vi "Measurement Logic.vi"(8 "error in":errorcluster, 9 "measurement configuration":T13={"double array in"=[3.4, 5.6], "double in"=1.2, "U32 array in"=[32, 33], "U32 in"=32, "U64 array in"=[64, 65], "U64 in"=64, "I32 array in"=[-32, -33], "I32 in"=-32, "I64 array in"=[-64, -65], "I64 in"=-64, "bool in"=TRUE, "string in"="Lorem ipsum dolor sit", "u32 color ring in"=1, "u32 animal enum in"=enum."Gopher"} {"u32 color ring in" items=["Red", "Green", "Blue"]}, 10 "measure call context in":refnum<class "Measure Call Context.lvclass">) -> (0 "Error Out":errorcluster, 2 "measure call context out":refnum<class "Measure Call Context.lvclass">, 3 "measurement results":T1)   [LabVIEW 2025, in "Automotive Vision.lvclass"]
doc: "Contains the core logic for executing the measurement."
uses:
  Automotive Vision.lvclass
  1487 HIHO GSE/Host/Common/Types/Packet Table.ctl
  <vilib>/Plug-In SDKs/Measurements/Measure Call Context/Measure Call Context.lvclass
  Measurement Configuration.ctl
  <instrlib>/FlexRIO/CSI-2/v2/FPGA/Types/GPIO Bank.ctl
  <vilib>/userDefined/Silver/nirio_resource_slv.ctl
  1487 HIHO GSE/Host/Acq/Types/CSI-2 Data Source.ctl
  1487 HIHO GSE/Host/Common/Types/Serial Channel Configuration.ctl
  <instrlib>/FlexRIO/CSI-2/v2/FPGA/Types/Display Parameters.ctl
  <instrlib>/FlexRIO/CSI-2/v2/Common/Types/LLP Data Type.ctl
  1487 HIHO GSE/Host/Common/Types/RAW Interpretation for Display.ctl
  Measurement Results.ctl
  <instrlib>/FlexRIO/CSI-2/v2/FPGA/Types/Timestamp ID.ctl
  1487 HIHO GSE/Host/Common/Types/GPIO Filter.ctl
  1487 HIHO GSE/FPGA/Common/Types/SerDes Identifier.ctl
  <vilib>/vision/Image Controls.llb/IMAQ Image.ctl
  <vilib>/Utility/miscctls.llb/LVRowAndColumnUnsignedTypeDef.ctl
  <instrlib>/FlexRIO/API/Host/v1/NI FlexRIO/API/Wait for PoC Safe to Disconnect Channels Array.vi
  <vilib>/FPGAPlugInAG/Dynamic/niLvFpga_Close_Dynamic.vi
  <extravilib>/ChannelInstances/Event Messenger-bool/Instantiate.vi
  <vilib>/rvi/interface/nirviCloseFPGA/nirviCloseFPGA.xnode
  Automotive Vision.lvclass/Automotive Vision.ctl
  1487 HIHO GSE/Host/Acq/GettingStarted_Acq_148X_Host.lvlib
  1487 HIHO GSE/Host/Common/GettingStarted_Common_148X_Host.lvlib
  <instrlib>/FlexRIO/API/Host/v1/NI FlexRIO API v1.lvlib
  <instrlib>/FlexRIO/CSI-2/v2/Common/NI CSI-2 API Common v2.lvlib
  <instrlib>/FlexRIO/CSI-2/v2/FPGA/NI CSI-2 API FPGA v2.lvlib
  1487 HIHO GSE/FPGA/Common/GettingStarted_Common_148X_FPGA.lvlib
panel:
  in  "Array":u32[](array[numeric])
  in  "Serial Channel (2nd Display)":fxp<+,3,3>
  in  "Serial Channel (1st Display)":fxp<+,3,3>
  in  "Configuration":T2(tab)
  in  "TDMS File Directory":path=path "C:/dev/hardware-validation/src/labview/auto-vision/Automotive Vision/1487 HIHO GSE/TDMS capture"
  in  "RIO Device":T3="PXI1Slot2"
  in  "Channel Configurations":T4[](array[typedef])=[{"Serial Channel"="SI1", "FPGA Display Parameters"={"virtual channel"=0.0, "payload data type"=enum."RAW 8", "frame skip count"=0, "line skip count"=0, "pixel skip count"=0.0}, "RAW Display Parameters"={"Interpretation"=enum."Bayer", "Bayer Parameters"={"Pattern"=3, "Algorithm"=0, "Red Gain"=1.0, "Green Gain"=1.0, "Blue Gain"=1.0}}}] {"RAW Display Parameters"."Bayer Parameters"."Blue Gain" min=0.0 max=3.99 step=0.1 format="%_4g"; "RAW Display Parameters"."Bayer Parameters"."Green Gain" min=0.0 max=3.99 step=0.1 format="%_4g"; "RAW Display Parameters"."Bayer Parameters"."Red Gain" min=0.0 max=3.99 step=0.1 format="%_4g"; "RAW Display Parameters"."Bayer Parameters"."Algorithm" items=["Bilinear", "VNG"]; "RAW Display Parameters"."Bayer Parameters"."Pattern" items=["GB", "GR", "BG", "RG"]}
  in  "CSI-2 Data Source":T8=1 items=["Raw", "Corrected"]
  in  "Configuration Script":path=path "C:/dev/hardware-validation/src/labview/auto-vision/Automotive Vision/1487 HIHO GSE/scripts/Image Receiver Scripts/9296A_RAW8.cpp"
  in  "Serial Input Active Lane Count":i32(ring)=4 items=["1 Lane"=1, "2 Lanes"=2, "4 Lanes"=4]
  in  "Reference Clock Frequency (Hz)":dbl=25000000.0 format="%#_6p"
  in  "Power Over Coax Source":i32(ring) items=["None", "Internal", "Auxiliary"]
  out "GPIO Bank Read":T9
  out "Power Over Coax Voltage (V)":dbl[](array[numeric]) format="%#.2pV"
  out "Power Over Coax Current (A)":dbl[](array[numeric]) format="%#.2pA"
  in  "Acquired Serial Input Channel Data":T10(tab)
  out "Source Rate (fps)(1st Display)":dbl
  out "Update Rate (fps)(1st Display)":dbl
  out "1st channel display":T11(plugin-control)
  out "Bytes Acquired (1st Channel)":i64 format="%#.6p"
  out "Source Rate (fps)(2nd Display)":dbl
  out "Update Rate (fps)(2nd Display)":dbl
  out "2nd channel display":T11(plugin-control)
  out "Acquired Packets (1st Channel)":T12
  out "Packets Logged (1st Channel)":i64
  out "Bytes Acquired (2nd Channel)":i64 format="%#.6p"
  out "Acquired Packets (2nd Channel)":T12
  out "Packets Logged (2nd Channel)":i64
  out "I2C Timestamps":T12
  out "GPIO Timestamps Waveform":digitalwaveform[](graph)
  out "Error Parsing GPIO Timestamps":bool
  out "Power Over Coax Source In Range":bool[](array[boolean])
  in  "Stop Acquisition":bool
  out "Acquisition In Progress":bool
  out "Acquisition Duration (s) 2":dbl format="%.1f"
  out "Acquisition Stopped":bool
  # "Resource Configuration"
  # "Data Output Configuration"
  # "Channel Configuration"
  # "Acquisition Configuration"
  # "First and Last Packet Select Configuration"
  # "Packet Filter Configuration"
  # "Power Over Coax Configuration"
  # "Clocking Configuration"
  # "I2C Timestamp Configuration"
  # "The timestamp filters listed correspond to the I2C traffic for a specific serial channel:\n\nUser24 = SI0\nUser25 = SI1\nUser26 = SI2\nUser27 = SI3\nUser28 = SI4\nUser29 = SI5\nUser30 = SI6\nUser31 = SI7"
  # "GPIO Configuration"
  # "* For additional packet viewing capability, use GettingStarted_Common_148X_Host.lvlib->TDMS File Viewer.vi"
  # "* For additional packet viewing capability, use GettingStarted_Common_148X_Host.lvlib->TDMS File Viewer.vi"
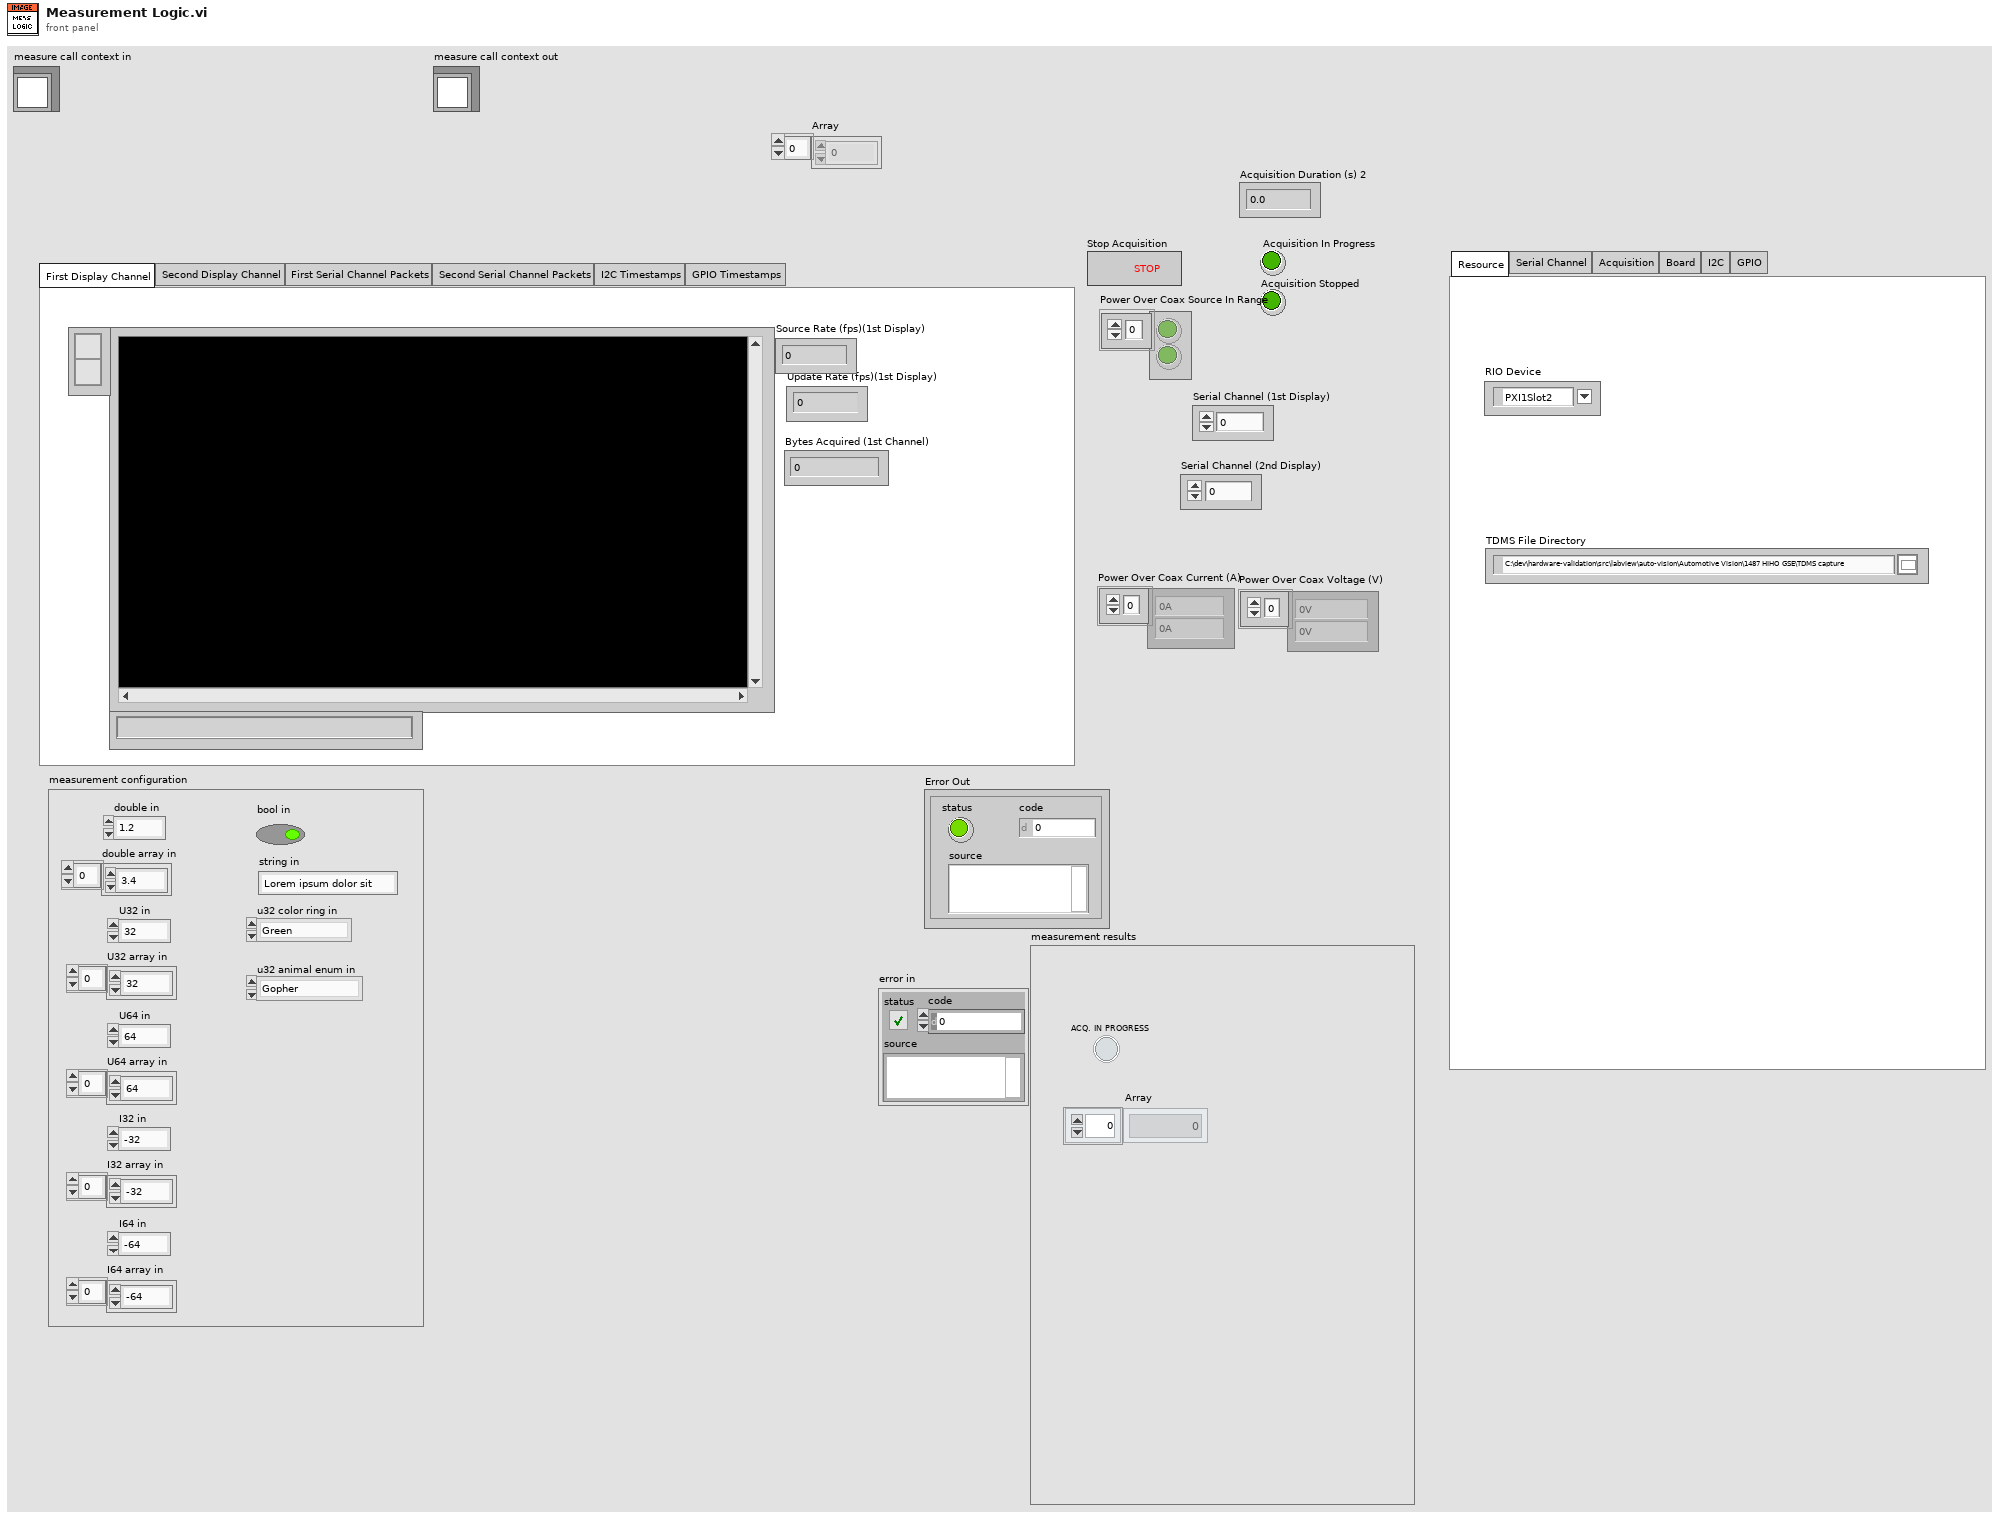
[diagram p1: front panel]
types:
  T1 = typedef "Automotive Vision.lvclass/Measurement Results.ctl" = cluster{"ACQ. IN PROGRESS":bool, "Array":u32[]}
  T2 = enum32{"Resource", "Serial Channel", "Acquisition", "Board", "I2C", "GPIO"}
  T3 = typedef "nirio_resource_slv.ctl" = tag
  T4 = typedef "GettingStarted_Common_148X_Host.lvlib/Serial Channel Configuration.ctl" = cluster{"Serial Channel":string, "FPGA Display Parameters":T5, "RAW Display Parameters":cluster{"Interpretation":T7, "Bayer Parameters":cluster{"Pattern":i32, "Algorithm":i32, "Red Gain":dbl, "Green Gain":dbl, "Blue Gain":dbl}}}
  T5 = typedef "NI CSI-2 API FPGA v2.lvlib/Display Parameters.ctl" = cluster{"virtual channel":fxp<+,4,4>, "payload data type":T6, "frame skip count":u16, "line skip count":u8, "pixel skip count":fxp<+,5,5>}
  T6 = typedef "NI CSI-2 API Common v2.lvlib/LLP Data Type.ctl" = enum8{"Frame Start", "Frame End", "Line Start", "Line End", "End of Transmission", "Reserved 0", "Reserved 1", "Reserved 2", "Generic Short Packet 1", "Generic Short Packet 2", "Generic Short Packet 3", "Generic Short Packet 4", "Generic Short Packet 5", "Generic Short Packet 6", "Generic Short Packet 7", "Generic Short Packet 8", "Null", "Blanking Data", "Embedded 8-bit non Image Data", "Generic Long Packet 1", "Generic Long Packet 2", "Generic Long Packet 3", "Generic Long Packet 4", "Reserved 3", "YUV420 8-bit", "YUV420 10-bit", "Legacy YUV420 8-bit", "Reserved 4", "YUV420 8-bit Chroma Shifted", "YUV420 10-bit Chroma Shifted", "YUV422 8-bit", "YUV422 10-bit", "RGB444", "RGB555", "RGB565", "RGB666", "RGB888", "Reserved 5", "Reserved 6", "RAW 24", "RAW 6", "RAW 7", "RAW 8", "RAW 10", "RAW 12", "RAW 14", "RAW 16", "RAW 20", "User Defined 8-bit Data 1", "User Defined 8-bit Data 2", "User Defined 8-bit Data 3", "User Defined 8-bit Data 4", "User Defined 8-bit Data 5", "User Defined 8-bit Data 6", "User Defined 8-bit Data 7", "User Defined 8-bit Data 8", "USL Command", "Reserved 7", "Reserved 8", "Reserved 9", "Reserved 10", "Reserved 11", "Reserved 12", "LRTE EPD Spacer"}
  T7 = typedef "GettingStarted_Common_148X_Host.lvlib/RAW Interpretation for Display.ctl" = enum16{"Grayscale", "Bayer", "RGB", "YUV422", "YUV420", "Legacy YUV420"}
  T8 = typedef "GettingStarted_Acq_148X_Host.lvlib/CSI-2 Data Source.ctl" = u16
  T9 = typedef "NI CSI-2 API FPGA v2.lvlib/GPIO Bank.ctl" = cluster{"GPIO 0":bool, "GPIO 1":bool, "GPIO 2":bool, "GPIO 3":bool, "GPIO 4":bool, "GPIO 5":bool, "GPIO 6":bool, "GPIO 7":bool, "GPIO 8":bool, "GPIO 9":bool, "GPIO 10":bool}
  T10 = enum32{"First Display Channel", "Second Display Channel", "First Serial Channel Packets", "Second Serial Channel Packets", "I2C Timestamps", "GPIO Timestamps"}
  T11 = typedef "IMAQ Image.ctl" = refnum<image>
  T12 = typedef "GettingStarted_Common_148X_Host.lvlib/Packet Table.ctl" = string[][]
  T13 = typedef "Automotive Vision.lvclass/Measurement Configuration.ctl" = cluster{"double array in":dbl[], "double in":dbl, "U32 array in":u32[], "U32 in":u32, "U64 array in":u64[], "U64 in":u64, "I32 array in":i32[], "I32 in":i32, "I64 array in":i64[], "I64 in":i64, "bool in":bool, "string in":string, "u32 color ring in":u32, "u32 animal enum in":enum32{"Rabbit", "Gopher", "Badger"}}
  T14 = typedef "GettingStarted_Common_148X_Host.lvlib/GPIO Filter.ctl" = cluster{"GPIO Bank":T15, "GPIO Number":i32}
  T15 = typedef "NI CSI-2 API FPGA v2.lvlib/Timestamp ID.ctl" = enum8{"SI0 LLP", "SI1 LLP", "SI2 LLP", "SI3 LLP", "SI4 LLP", "SI5 LLP", "SI6 LLP", "SI7 LLP", "SO0 LLP", "SO1 LLP", "SO2 LLP", "SO3 LLP", "SO4 LLP", "SO5 LLP", "SO6 LLP", "SO7 LLP", "Ser0 GPIO Bank", "Ser1 GPIO Bank", "Ser2 GPIO Bank", "Ser3 GPIO Bank", "Ser4 GPIO Bank", "Ser5 GPIO Bank", "Ser6 GPIO Bank", "Ser7 GPIO Bank", "Des0 GPIO Bank", "Des1 GPIO Bank", "Des2 GPIO Bank", "Des3 GPIO Bank", "Des4 GPIO Bank", "Des5 GPIO Bank", "Des6 GPIO Bank", "Des7 GPIO Bank", "User0", "User1", "User2", "User3", "User4", "User5", "User6", "User7", "User8", "User9", "User10", "User11", "User12", "User13", "User14", "User15", "User16", "User17", "User18", "User19", "User20", "User21", "User22", "User23", "User24", "User25", "User26", "User27", "User28", "User29", "User30", "User31"}
  T16 = typedef "LVRowAndColumnUnsignedTypeDef.ctl" = cluster{"Row":u32, "Column":u32}
  T17 = typedef "GettingStarted_Common_148X_Host.lvlib/Serial Channel Display Parameters.ctl" = cluster{"images":cluster{"grayscale":T11, "color":T11}, "RAW parameters":cluster{"interpretation":T7, "bayer parameters":cluster{"pattern":i32, "algorithm":i32, "red gain":dbl, "green gain":dbl, "blue gain":dbl}}}
  T18 = cluster{"Source Rate (fps)(1st Display)":refnum<vi>, "Update Rate (fps)(1st Display)":refnum<vi>}
  T19 = cluster{"Source Rate (fps)(2nd Display)":refnum<vi>, "Update Rate (fps)(2nd Display)":refnum<vi>}
  T20 = cluster{"Source Rate (fps)(2nd Display)":refnum<vi>, "Update Rate (fps)(2nd Display)":refnum<vi>}[]
  T21 = typedef "GettingStarted_Common_148X_FPGA.lvlib/SerDes Identifier.ctl" = enum8{"None", "SI 0 Deserializer", "SI 1 Deserializer", "SI 2 Deserializer", "SI 3 Deserializer", "SI 4 Deserializer", "SI 5 Deserializer", "SI 6 Deserializer", "SI 7 Deserializer", "SO 0 Serializer", "SO 1 Serializer", "SO 2 Serializer", "SO 3 Serializer", "SO 4 Serializer", "SO 5 Serializer", "SO 6 Serializer", "SO 7 Serializer", "SI 0 SI 1 Deserializer", "SI 2 SI 3 Deserializer", "SI 4 SI 5 Deserializer", "SI 6 SI 7 Deserializer"}
  T22 = typedef "Event Messenger-bool.lvlib/))Channel.ctl" = refnum<queue>
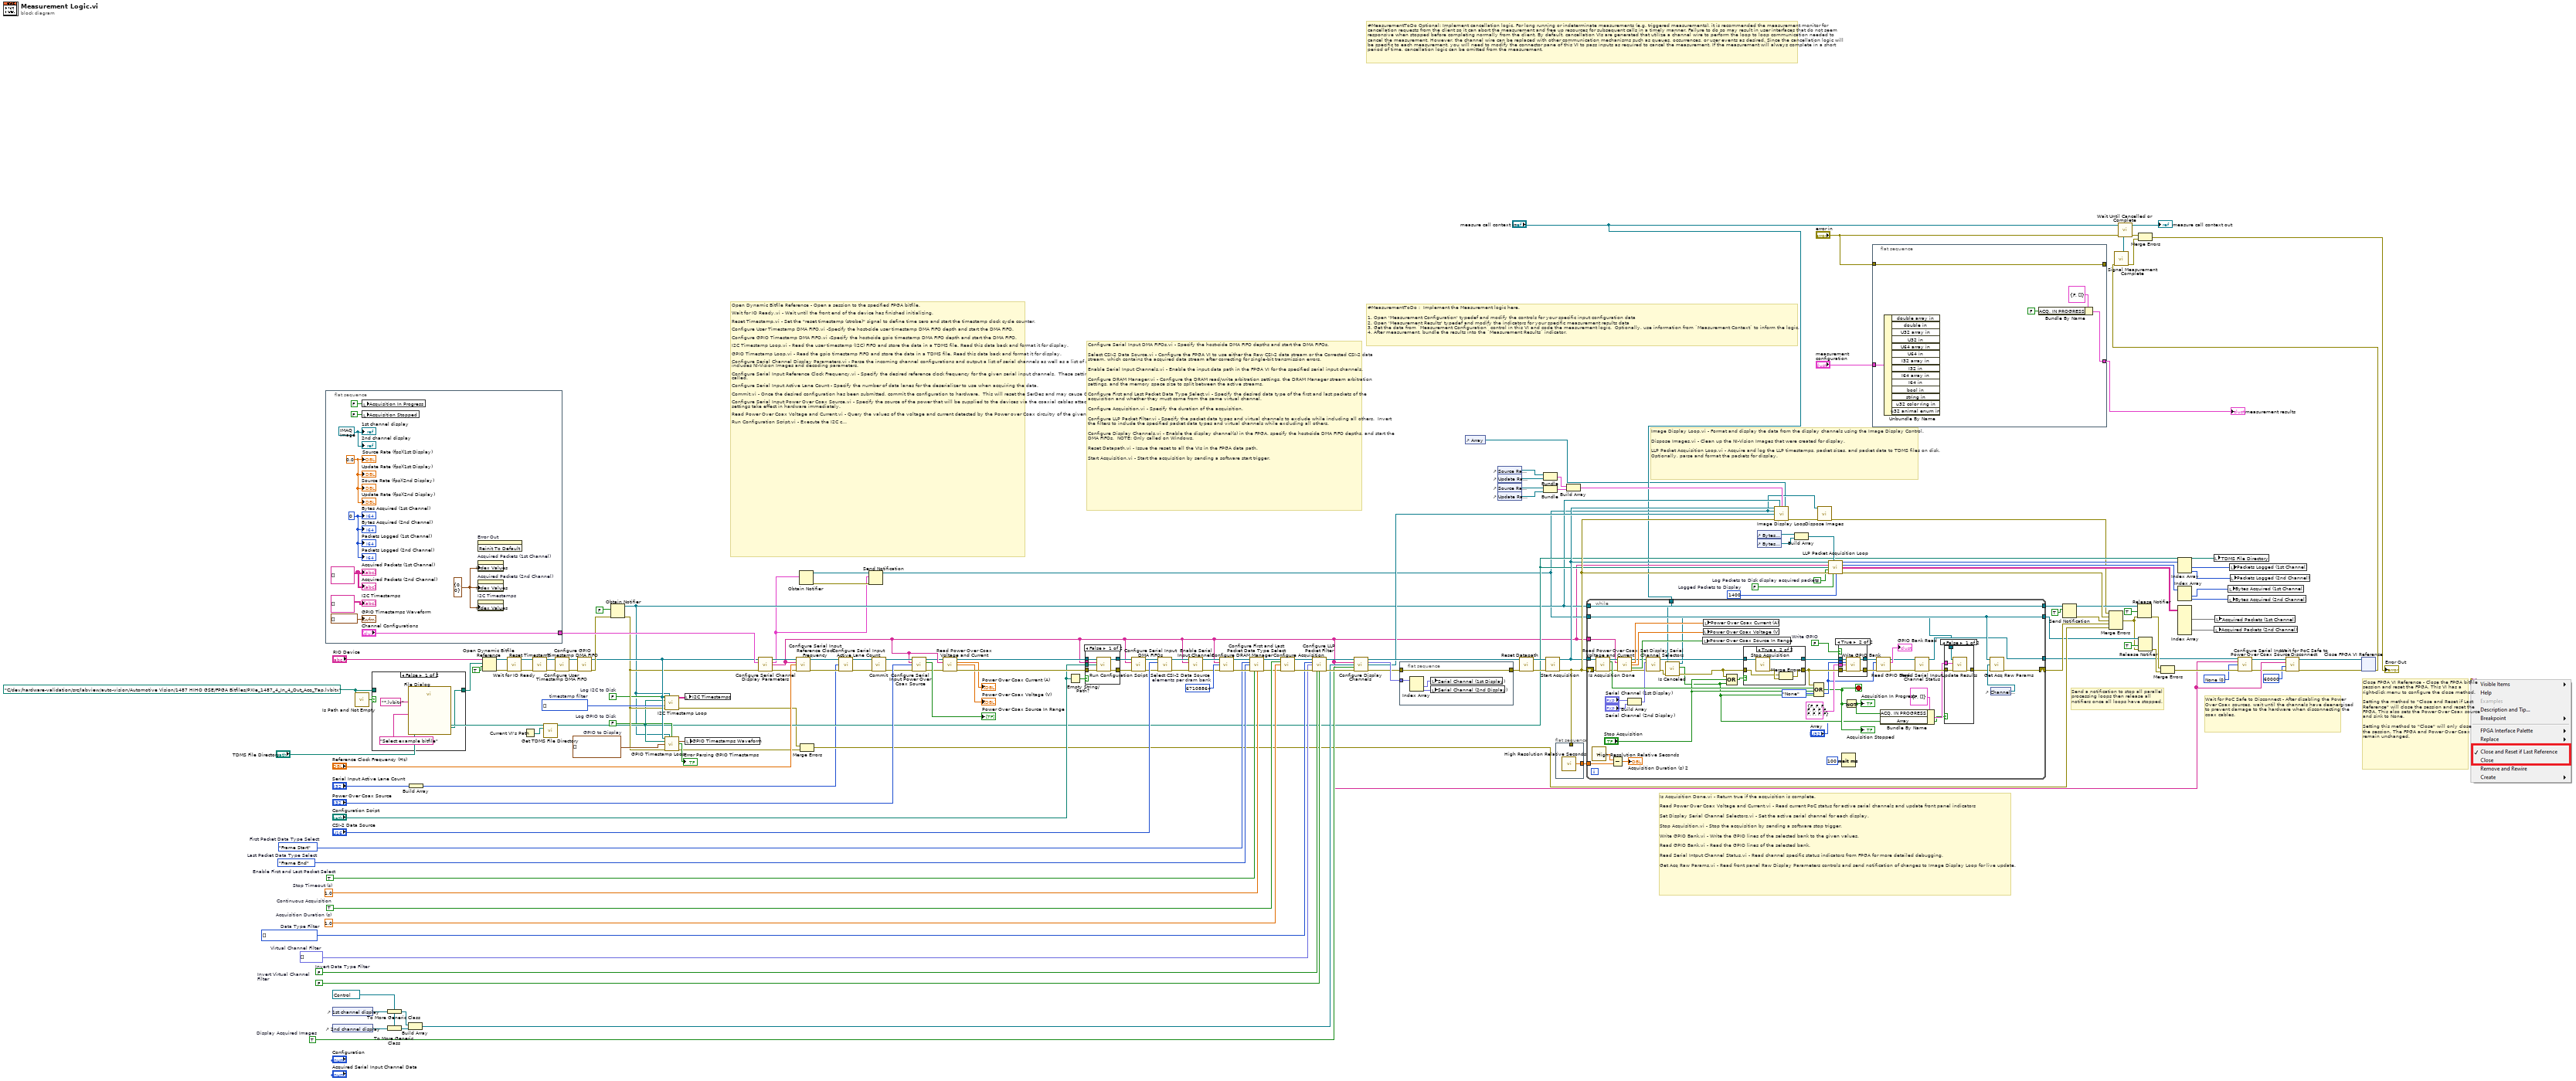
[diagram p0: block diagram]
diagram:
  w35 = i64 1400  # Logged Packets to Display
  w74 = FALSE  # Log Packets to Disk
  w123 = FALSE  # Invert Virtual Channel Filter
  w124 = FALSE  # Invert Data Type Filter
  w130 = fxp<+,4,4>[] []  # Virtual Channel Filter
  w45 = T14[] []  # GPIO to Display
  w41 = FALSE  # Log GPIO to Disk
  w44 = T15[] [] items=["SI0 LLP", "SI1 LLP", "SI2 LLP", "SI3 LLP", "SI4 LLP", "SI5 LLP", "SI6 LLP", "SI7 LLP", "SO0 LLP", "SO1 LLP", "SO2 LLP", "SO3 LLP", "SO4 LLP", "SO5 LLP", "SO6 LLP", "SO7 LLP", "Ser0 GPIO Bank", "Ser1 GPIO Bank", "Ser2 GPIO Bank", "Ser3 GPIO Bank", "Ser4 GPIO Bank", "Ser5 GPIO Bank", "Ser6 GPIO Bank", "Ser7 GPIO Bank", "Des0 GPIO Bank", "Des1 GPIO Bank", "Des2 GPIO Bank", "Des3 GPIO Bank", "Des4 GPIO Bank", "Des5 GPIO Bank", "Des6 GPIO Bank", "Des7 GPIO Bank", "User0", "User1", "User2", "User3", "User4", "User5", "User6", "User7", "User8", "User9", "User10", "User11", "User12", "User13", "User14", "User15", "User16", "User17", "User18", "User19", "User20", "User21", "User22", "User23", "User24", "User25", "User26", "User27", "User28", "User29", "User30", "User31"]  # timestamp filter
  w42 = FALSE  # Log I2C to Disk
  w69 = TRUE  # Display Acquired Images
  w137 = T6[] [] items=["Frame Start", "Frame End", "Line Start", "Line End", "End of Transmission", "Reserved 0", "Reserved 1", "Reserved 2", "Generic Short Packet 1", "Generic Short Packet 2", "Generic Short Packet 3", "Generic Short Packet 4", "Generic Short Packet 5", "Generic Short Packet 6", "Generic Short Packet 7", "Generic Short Packet 8", "Null", "Blanking Data", "Embedded 8-bit non Image Data", "Generic Long Packet 1", "Generic Long Packet 2", "Generic Long Packet 3", "Generic Long Packet 4", "Reserved 3", "YUV420 8-bit", "YUV420 10-bit", "Legacy YUV420 8-bit", "Reserved 4", "YUV420 8-bit Chroma Shifted", "YUV420 10-bit Chroma Shifted", "YUV422 8-bit", "YUV422 10-bit", "RGB444", "RGB555", "RGB565", "RGB666", "RGB888", "Reserved 5", "Reserved 6", "RAW 24", "RAW 6", "RAW 7", "RAW 8", "RAW 10", "RAW 12", "RAW 14", "RAW 16", "RAW 20", "User Defined 8-bit Data 1", "User Defined 8-bit Data 2", "User Defined 8-bit Data 3", "User Defined 8-bit Data 4", "User Defined 8-bit Data 5", "User Defined 8-bit Data 6", "User Defined 8-bit Data 7", "User Defined 8-bit Data 8", "USL Command", "Reserved 7", "Reserved 8", "Reserved 9", "Reserved 10", "Reserved 11", "Reserved 12", "LRTE EPD Spacer"]  # Data Type Filter
  w140 = 1.0  # Acquisition Duration (s)
  w146 = TRUE  # Continuous Acquisition
  w112 = 1.0  # Stop Timeout (s)
  w113 = TRUE  # Enable First and Last Packet Select
  w110 = LLP_Data_Type."Frame End"  # Last Packet Data Type Select
  w111 = LLP_Data_Type."Frame Start"  # First Packet Data Type Select
  w135 = path "C:/dev/hardware-validation/src/labview/auto-vision/Automotive Vision/1487 HIHO GSE/FPGA Bitfiles/PXIe_1487_4_In_4_Out_Acq_Tap.lvbitx" ("Bitfile Path")
  w9 = 0 items=["None", "Internal", "Auxiliary"] ("power over coax source")
  w36 = TRUE  # display acquired packets
  w87 = refnum<vi> refnum ("image display reference")
  w152 = u32 67108864  # elements per dram bank
  # "Wait for PoC Safe to Disconnect - After disabling the Power Over Coax sources, wait until the channels have deenergized to prevent damage to the hardware when disconnecting the coax cables."
  # "Send a notification to stop all parallel processing loops then release all notifiers once all loops have stopped."
  # "Image Display Loop.vi - Format and display the data from the display channels using the Image Display Control.   \n\nDispose Images.vi - Clean up the NI-Vision Images that were created for display.\n\nLLP Packet Acquisition Loop.vi - Acquire and log the LLP timestamps, packet sizes, and packet data to TDMS files on disk.  Optionally, parse and format the packets for display."
  # "Configure Serial Input DMA FIFOs.vi - Specify the host-side DMA FIFO depths and start the DMA FIFOs.\n\nSelect CSI-2 Data Source.vi - Configure the FPGA VI to use either the Raw CSI-2 data stream or the Corrected CSI-2 data stream, which contains the acquired data stream after correcting for single-bit transmission errors.\n\nEnable Serial Input Channels.vi - Enable the input data path in the FPGA VI for the specified serial input channels.\n\nConfigure DRAM Manager.vi - Configure the DRAM read/write arbitration settings, the DRAM Manager stream arbitration settings, and the memory space size to split between the active streams.\n\nConfigure First and Last Packet Data Type Select.vi - Specify the desired data type of the first and last packets of the acquisition and whether they must come from the same virtual channel.\n\nConfigure Acquisition.vi - Specify the duration of the acquisition.\n\nConfigure LLP Packet Filter.vi - Specify the packet data types and virtual channels to exclude while including all others.  Invert the filters to include the specified packet data types and virtual channels while excluding all others.\n\nConfigure Display Channels.vi - Enable the display channel(s) in the FPGA, specify the host-side DMA FIFO depths, and start the DMA FIFOs.  NOTE: Only called on Windows. \n\nReset Datapath.vi - Issue the reset to all the VIs in the FPGA data path.\n\nStart Acquisition.vi - Start the acquisition by sending a software start trigger."
  # "Close FPGA VI Reference - Close the FPGA bitfile session and reset the FPGA. This VI has a right-click menu to configure the close method. \n\nSetting the method to \"Close and Reset if Last Reference\" will close the session and reset the FPGA. This also sets the Power Over Coax source and sink to None.\n\nSetting this method to \"Close\" will only close the session. The FPGA and Power Over Coax remain unchanged."
  # "Open Dynamic Bitfile Reference - Open a session to the specified FPGA bitfile.\n\nWait for IO Ready.vi - Wait until the front end of the device has finished initializing.\n\nReset Timestamp.vi - Set the \"reset timestamp (strobe)\" signal to define time zero and start the timestamp clock cycle counter.\n\nConfigure User Timestamp DMA FIFO.vi -Specify the host-side user timestamp DMA FIFO depth and start the DMA FIFO.\n\nConfigure GPIO Timestamp DMA FIFO.vi -Specify the host-side gpio timestamp DMA FIFO depth and start the DMA FIFO.\n\nI2C Timestamp Loop.vi - Read the user timestamp (I2C) FIFO and store the data in a TDMS file. Read this data back and format it for display.\n\nGPIO Timestamp Loop.vi - Read the gpio timestamp FIFO and store the data in a TDMS file. Read this data back and format it for display.\n\nConfigure Serial Channel Display Parameters.vi - Parse the incoming channel configurations and output a list of serial channels as well as a list of serial channel display parameters, which includes NI-Vision Images and decoding parameters.\n\nConfigure Serial Input Reference Clock Frequency.vi - Specify the desired reference clock frequency for the given serial input channels.  These settings do not take effect until Commit.vi is called.\n\nConfigure Serial Input Active Lane Count - Specify the number of data lanes for the deserializer to use when acquiring the data. \n\nCommit.vi - Once the desired configuration has been submitted, commit the configuration to hardware.  This will reset the SerDes and may cause GPIO lines to toggle. \n\nConfigure Serial Input Power Over Coax Source.vi - Specify the source of the power that will be supplied to the devices via the coaxial cables attached to the given serial input channels.  These settings take effect in hardware immediately.\n\nRead Power Over Coax Voltage and Current.vi - Query the values of the voltage and current detected by the Power over Coax circuitry of the given serial channels.\n\nRun Configuration Script.vi - Execute the I2C commands in the specified script file for the given serial channels.  The script is used to configure the serializer, deserializer, or other I2C slave device, such as the image sensor."
  # "Is Acquisition Done.vi - Return true if the acquisition is complete.\n\nRead Power Over Coax Voltage and Current.vi - Read current PoC status for active serial channels and update front panel indicators \n\nSet Display Serial Channel Selectors.vi - Set the active serial channel for each display.\n\nStop Acquisition.vi - Stop the acquisition by sending a software stop trigger.\n\nWrite GPIO Bank.vi - Write the GPIO lines of the selected bank to the given values.\n\nRead GPIO Bank.vi - Read the GPIO lines of the selected bank.\n\nRead Serial Intput Channel Status.vi - Read channel specific status indicators from FPGA for more detailed debugging.\n\nGet Acq Raw Params.vi - Read front panel Raw Display Parameters controls and send notification of changes to Image Display Loop for live update."
  # "#MeasurementToDo Optional: Implement cancellation logic. For long running or indeterminate measurements (e.g. triggered measurements), it is recommended the measurement monitor for cancellation requests from the client so it can abort the measurement and free up resources for subsequent calls in a timely manner. Failure to do so may result in user interfaces that do not seem responsive when stopped before completing normally from the client. By default, cancellation VIs are generated that utilize a channel wire to perform the loop to loop communication needed to cancel the measurement. However, the channel wire can be replaced with other communication mechanisms such as queues, occurrences, or user events as desired. Since the cancellation logic will be specific to each measurement, you will need to modify the connector pane of this VI to pass inputs as required to cancel the measurement. If the measurement will always complete in a short period of time, cancellation logic can be omitted from the measurement."
  # "#MeasurementToDo :  Implement the Measurement logic here.\n\n1. Open 'Measurement Configuration' typedef and modify the controls for your specific input configuration data\n2. Open 'Measurement Results' typedef and modify the indicators for your specific measurement results data\n3. Get the data from `Measurement Configuration` control in this VI and code the measurement logic.  Optionally, use information from `Measurement Context` to inform the logic.\n4. After measurement, bundle the results into the `Measurement Results` indicator."
  n1 = flat-sequence {
    tunnel: ["Channel Configurations"] -> w101
    frame #0 {
      w159 = T16 {"Row"=0, "Column"=0} ("Index Values")
      w166 = T12 [] ("Acquired Packets (1st Channel)")
      w162 = 0 ("Number of Packets Acquired (1st Channel)")
      w165 = 0.0 ("display fps (2nd display)")
      w168 = T11 refnum ("first channel display")
      n2 = local write "Acquisition In Progress"(FALSE ("Acquisition In Progress")) -> ()
      n3 = local write "Acquisition Stopped"(FALSE ("Acquisition Stopped")) -> ()
      n4 = invoke on="Error Out" class="Clust (strict)" method="Reinit To Default"() -> ()  [unwired: 3 in, 3 out]
      n5 = property on="Acquired Packets (1st Channel)" class="Tbl (strict)"("Index Values"=w159) -> ()  [unwired: 2 in, 2 out]
      n6 = property on="Acquired Packets (2nd Channel)" class="Tbl (strict)"("Index Values"=w159) -> ()  [unwired: 2 in, 2 out]
      n7 = property on="I2C Timestamps" class="Tbl (strict)"("Index Values"=w159) -> ()  [unwired: 2 in, 2 out]
      "1st channel display" <- w168
      "2nd channel display" <- w168
      "Update Rate (fps)(1st Display)" <- w165
      "Update Rate (fps)(2nd Display)" <- w165
      "Acquired Packets (1st Channel)" <- w166
      "Packets Logged (1st Channel)" <- w162
      "Acquired Packets (2nd Channel)" <- w166
      "Packets Logged (2nd Channel)" <- w162
      "Source Rate (fps)(1st Display)" <- w165
      "Source Rate (fps)(2nd Display)" <- w165
      "GPIO Timestamps Waveform" <- digitalwaveform[] [] ("GPIO Timestamps Waveform")
      "I2C Timestamps" <- T12 [] ("I2C Timestamps 2")
      "Bytes Acquired (1st Channel)" <- w162
      "Bytes Acquired (2nd Channel)" <- w162
    }
  }
  n8 = control-ref of="1st channel display"() -> (w98:refnum<vi>)
  n9 = control-ref of="2nd channel display"() -> (w96:refnum<vi>)
  n10 = call <vilib>:"Is Path and Not Empty.vi"("path"=w135) -> ("Is Path and Not Empty?"=w134:bool)  [unwired: 4 in]
  n11 = case shown="False" w134 {
    tunnel: w135 -> [_ w172]
    tunnel: [w170 w172] -> w133
    frame False {
      n12 = call "File Dialog"("prompt"="Select example bitfile", "pattern (all files)"="*.lvbitx") -> ("selected path"=w170:path)  [unwired: 10 in, 3 out]
    }
    frame True {
    }
  }
  n13 = To More Generic Class(target class=w87, reference=w98) -> (generic class reference=w97:refnum<vi>)
  n14 = To More Generic Class(target class=w87, reference=w96) -> (generic class reference=w95:refnum<vi>)
  n15 = Build Array(w97, w95) -> (w93:refnum<vi>[])
  n16 = Build Array("Serial Input Active Lane Count") -> (w27:i32[])
  n17 = Open Dynamic Bitfile Reference(0:"RIO Device", 1:w133, 2:TRUE ("Run When Loaded")) -> (5:w131:refnum<k20>, 8:w132:errorcluster)  [unwired: 2 in]
  n18 = call <instrlib>:"Wait for IO Ready.vi"("fpga interface in"=w131, "error in"=w132) -> ("fpga interface out"=w65:refnum<k20>, "error out"=w66:errorcluster)  [unwired: 10 in, 2 out]
  n19 = Current VI's Path() -> (path=w105:path)
  n20 = call "Reset Timestamp.vi"("fpga interface in"=w65, "error in (no error)"=w66) -> ("fpga interface out"=w55:refnum<k20>, "error out"=w54:errorcluster)  [unwired: 12 in]
  n21 = call "Get TDMS File Directory.vi"("tdms file directory in"="TDMS File Directory", "calling vi path"=w105) -> ("tdms file directory out"=w40:path)  [unwired: 13 in]
  n22 = call "Configure User Timestamp DMA FIFO.vi"("fpga interface in"=w55, "error in (no error)"=w54) -> ("fpga interface out"=w53:refnum<k20>, "error out"=w52:errorcluster)  [unwired: 12 in]
  n23 = call "Configure GPIO Timestamp DMA FIFO.vi"("fpga interface in"=w53, "error in (no error)"=w52) -> ("fpga interface out"=w49:refnum<k20>, "error out"=w51:errorcluster)  [unwired: 12 in]
  n24 = Obtain Notifier(notification data type=FALSE ("result"), error in (no error)=w51) -> (notifier out=w26:refnum<notifier>, error out=w43:errorcluster)  [unwired: 2 in, 1 out]
  n25 = call "I2C Timestamp Loop.vi"("fpga interface in"=w49, "'stop' notifier"=w26, "log i2c to disk"=w42, "tdms file directory"=w40, "timestamp filter"=w44, "error in (no error)"=w43) -> ("i2c data"=w48:string[][], "error out"=w38:errorcluster)  [unwired: 8 in]
  n26 = call "GPIO Timestamp Loop.vi"("fpga interface in"=w49, "'stop' notifier"=w26, "log gpio to disk"=w41, "tdms file directory"=w40, "gpio to display"=w45, "error in (no error)"=w43) -> ("gpio timestamps waveform"=w47:digitalwaveform[], "error parsing gpio timestamps"=→"Error Parsing GPIO Timestamps":bool, "error out"=w37:errorcluster)  [unwired: 7 in]
  n27 = local write "I2C Timestamps"(w48) -> ()
  n28 = local write "GPIO Timestamps Waveform"(w47) -> ()
  n29 = call "Configure Serial Channel Display Parameters.vi"("fpga interface in"=w49, "serial channel configurations"=w101, "error in (no error)"=w43) -> ("fpga interface out"=w100:refnum<k20>, "serial channel display parameters"=w23:T17[], "serial channels"=w12:string[], "error out"=w99:errorcluster)  [unwired: 9 in]
  n30 = call "Configure Serial Input Reference Clock Frequency.vi"("fpga interface in"=w100, "serial input channels"=w12, "serial input reference clock frequency (Hz)"="Reference Clock Frequency (Hz)", "error in (no error)"=w99) -> ("fpga interface out"=w32:refnum<k20>, "error out"=w31:errorcluster)  [unwired: 10 in]
  n31 = Obtain Notifier(notification data type=w23) -> (notifier out=w25:refnum<notifier>, error out=w24:errorcluster)  [unwired: 3 in, 1 out]
  n32 = Merge Errors(w38, w37) -> (w33:errorcluster)
  n33 = call "Configure Serial Input Active Lane Count.vi"("fpga interface in"=w32, "serial input active lane counts"=w27, "error in (no error)"=w31) -> ("fpga interface out"=w30:refnum<k20>, "error out"=w29:errorcluster)  [unwired: 11 in]
  n34 = Send Notification(notification=w23, notifier=w25, error in (no error)=w24) -> (notifier out=w22:refnum<notifier>)  [unwired: 1 out]
  n35 = call <instrlib>:"Commit.vi"("fpga interface in"=w30, "error in"=w29) -> ("fpga interface out"=w138:refnum<k20>, "error out"=w139:errorcluster)  [unwired: 12 in]
  n36 = call "Configure Serial Input Power Over Coax Source.vi"("fpga interface in"=w138, "serial input channels"=w12, "power over coax source"="Power Over Coax Source", "error in (no error)"=w139) -> ("fpga interface out"=w10:refnum<k20>, "power over coax source in range"=→"Power Over Coax Source In Range":bool[], "error out"=w11:errorcluster)  [unwired: 9 in]
  n37 = call "Read Power Over Coax Voltage and Current.vi"("fpga interface in"=w10, "serial channels"=w12, "error in (no error)"=w11) -> ("fpga interface out"=w128:refnum<k20>, "current (A)"=→"Power Over Coax Current (A)":dbl[], "voltage (V)"=→"Power Over Coax Voltage (V)":dbl[], "error out"=w129:errorcluster)  [unwired: 8 in, 1 out]
  n38 = Empty String/Path?(string/path="Configuration Script") -> (empty?=w68:bool)
  n39 = case shown="False" w68 {
    tunnel: [w178 w179] -> w150
    tunnel: [w177 w180] -> w142
    tunnel: w129 -> [w176 w179]
    tunnel: w128 -> [w175 w180]
    tunnel: w12 -> [w174 _]
    tunnel: "Configuration Script" -> [w173 _]
    frame False {
      n40 = call "Run Configuration Script.vi"("fpga interface in"=w175, "serial channels"=w174, "configuration script"=w173, "error in (no error)"=w176) -> ("fpga interface out"=w177:refnum<k20>, "error out"=w178:errorcluster)  [unwired: 10 in]
    }
    frame True {
    }
  }
  n41 = call "Configure Serial Input DMA FIFOs.vi"("fpga interface in"=w142, "serial channels"=w12, "error in (no error)"=w150) -> ("fpga interface out"=w121:refnum<k20>, "error out"=w118:errorcluster)  [unwired: 11 in]
  n42 = call "Select CSI-2 Data Source.vi"("fpga interface in"=w121, "csi-2 data source"="CSI-2 Data Source", "error in (no error)"=w118) -> ("fpga interface out"=w120:refnum<k20>, "error out"=w119:errorcluster)  [unwired: 11 in]
  n43 = call "Enable Serial Input Channels.vi"("fpga interface in"=w120, "serial input channels"=w12, "error in (no error)"=w119) -> ("fpga interface out"=w141:refnum<k20>, "error out"=w151:errorcluster)  [unwired: 11 in]
  n44 = call "Configure DRAM Manager.vi"("fpga interface in"=w141, "serial channels"=w12, "elements per dram bank"=w152, "error in (no error)"=w151) -> ("fpga interface out"=w114:refnum<k20>, "error out"=w117:errorcluster)  [unwired: 10 in]
  n45 = call "Configure First and Last Packet Data Type Select.vi"("fpga interface in"=w114, "first packet data type select"=w111, "last packet data type select"=w110, "error in (no error)"=w117, "enable first and last packet select"=w113, "stop timeout (s)"=w112) -> ("fpga interface out"=w115:refnum<k20>, "error out"=w116:errorcluster)  [unwired: 8 in]
  n46 = call "Configure Acquisition.vi"("fpga interface in"=w115, "continuous acquisition (T)"=w146, "acquisition duration (s)"=w140, "error in (no error)"=w116) -> ("fpga interface out"=w147:refnum<k20>, "error out"=w148:errorcluster)  [unwired: 10 in]
  n47 = call "Configure LLP Packet Filter.vi"("fpga interface in"=w147, "data type filter"=w137, "virtual channel filter"=w130, "error in (no error)"=w148, "invert data type filter"=w124, "invert virtual channel filter"=w123) -> ("fpga interface out"=w102:refnum<k20>, "error out"=w94:errorcluster)  [unwired: 8 in]
  n48 = call "Configure Display Channels.vi"("fpga interface in"=w102, "serial channels"=w12, "display references in"=w93, "enable image display"=w69, "error in (no error)"=w94) -> ("fpga interface out"=w92:refnum<k20>, "display serial channels"=w91:fxp<+,3,3>[], "display references out"=w88:refnum<vi>[], "error out"=w90:errorcluster)  [unwired: 7 in]
  n49 = flat-sequence {
    tunnel: w91 -> [w182]
    tunnel: w90 -> [w181]
    tunnel: [w181] -> w89
    frame #0 {
      n50 = Index Array(array=w182) -> (element #1=w184:fxp<+,3,3>, element #2=w183:fxp<+,3,3>)  [unwired: 2 in]
      n51 = local write "Serial Channel (1st Display)"(w184) -> ()
      n52 = local write "Serial Channel (2nd Display)"(w183) -> ()
    }
  }
  n53 = control-ref of="Array"() -> (w1:refnum<vi>)
  n54 = control-ref of="Source Rate (fps)(1st Display)"() -> (w80:refnum<vi>)
  n55 = control-ref of="Update Rate (fps)(1st Display)"() -> (w81:refnum<vi>)
  n56 = control-ref of="Source Rate (fps)(2nd Display)"() -> (w79:refnum<vi>)
  n57 = control-ref of="Update Rate (fps)(2nd Display)"() -> (w78:refnum<vi>)
  n58 = call "Reset Datapath.vi"("fpga interface in"=w92, "error in (no error)"=w89) -> ("fpga interface out"=w149:refnum<k20>, "error out"=w50:errorcluster)  [unwired: 12 in]
  n59 = Bundle("Source Rate (fps)(1st Display)"=w80, "Update Rate (fps)(1st Display)"=w81) -> (w77:T18)  [unwired: 1 in]
  n60 = Bundle("Source Rate (fps)(2nd Display)"=w79, "Update Rate (fps)(2nd Display)"=w78) -> (w76:T19)  [unwired: 1 in]
  n61 = call "Start Acquisition.vi"("fpga interface in"=w149, "error in (no error)"=w50) -> ("fpga interface out"=w63:refnum<k20>, "error out"=w64:errorcluster)  [unwired: 12 in]
  n62 = flat-sequence {
    tunnel: [w185] -> w107
    tunnel: w64 -> [_]
    frame #0 {
      n63 = call <vilib>:"High Resolution Relative Seconds.vi"() -> ("relative seconds"=w185:dbl)
    }
  }
  n64 = Build Array(w77, w76) -> (w75:T20)
  n65 = while {
    shift-right: [w203] -> w34
    shift-left: w64 -> [w205]
    tunnel: w63 -> [w217]
    tunnel: w12 -> [w229]
    tunnel: w107 -> [w224]
    tunnel: w26 -> [w204]
    tunnel: [w204] -> w60
    tunnel: w22 -> [w201]
    tunnel: [w198] -> w16
    tunnel: [w201] -> w20
    tunnel: "measure call context in" -> [w195]
    stop <- w206 stop-if-true
    w209 = FALSE  # Write GPIO
    w208 = SerDes_Identifier."None" ("GPIO Bank Select")
    n66 = call <vilib>:"High Resolution Relative Seconds.vi"() -> ("relative seconds"=w225:dbl)
    n67 = call "Is Acquisition Done.vi"("fpga interface in"=w217, "error in (no error)"=w205) -> ("fpga interface out"=w230:refnum<k20>, "acquisition done"=w233:bool, "error out"=w231:errorcluster)  [unwired: 11 in]
    n68 = Subtract(x=w225, y=w224) -> (x-y=→"Acquisition Duration (s) 2":dbl)
    n69 = call "Read Power Over Coax Voltage and Current.vi"("fpga interface in"=w230, "serial channels"=w229, "error in (no error)"=w231) -> ("fpga interface out"=w219:refnum<k20>, "current (A)"=w228:dbl[], "voltage (V)"=w226:dbl[], "in range"=w227:bool[], "error out"=w218:errorcluster)  [unwired: 8 in]
    n70 = Build Array("Serial Channel (1st Display)", "Serial Channel (2nd Display)") -> (w220:fxp<+,3,3>[])
    n71 = call "Set Display Serial Channel Selectors.vi"("fpga interface in"=w219, "display serial channel selectors"=w220, "error in (no error)"=w218) -> ("fpga interface out"=w196:refnum<k20>, "error out"=w197:errorcluster)  [unwired: 11 in]
    n72 = call <vilib>:"Is Canceled.vi"("error in"=w197, "measure call context in"=w195) -> ("error out"=w188:errorcluster, "is canceled?"=w187:bool, "measure call context out"=w191:refnum<class "Measure Call Context.lvclass">)  [unwired: 7 in]
    n73 = local write "Power Over Coax Source In Range"(w227) -> ()
    n74 = local write "Power Over Coax Voltage (V)"(w226) -> ()
    n75 = local write "Power Over Coax Current (A)"(w228) -> ()
    n76 = Compound Arithmetic op=OR(w188, "Stop Acquisition", w187) -> (w216:bool)
    n77 = case shown="True" w216 {
      tunnel: [w248 w250] -> w214
      tunnel: w188 -> [w248 w249]
      tunnel: [w247 w252] -> w215
      tunnel: w196 -> [w247 w251]
      frame False {
      }
      frame True {
        n78 = call "Stop Acquisition.vi"("fpga interface in"=w251) -> ("fpga interface out"=w252:refnum<k20>, "error out"=w253:errorcluster)  [unwired: 13 in]
        n79 = Merge Errors(w249, w253) -> (w250:errorcluster)
      }
    }
    n80 = Compound Arithmetic op=OR(w214, w233, "Stop Acquisition", w187) -> (w206:bool)
    "Acquisition Stopped" <- w206
    n81 = case shown="True" w209 {
      tunnel: w215 -> [w240 w246]
      tunnel: w214 -> [w239 w245]
      tunnel: T9 {"GPIO 0"=FALSE, "GPIO 1"=FALSE, "GPIO 2"=FALSE, "GPIO 3"=FALSE, "GPIO 4"=FALSE, "GPIO 5"=FALSE, "GPIO 6"=FALSE, "GPIO 7"=FALSE, "GPIO 8"=FALSE, "GPIO 9"=FALSE, "GPIO 10"=FALSE} ("GPIO Bank Write") -> [_ w244]
      tunnel: [w240 w243] -> w212
      tunnel: [w239 w242] -> w211
      tunnel: w208 -> [_ w241]
      frame False {
      }
      frame True {
        n82 = call "Write GPIO Bank.vi"("fpga interface in"=w246, "gpio bank select"=w241, "gpio bank output"=w244, "error in (no error)"=w245) -> ("fpga interface out"=w243:refnum<k20>, "error out"=w242:errorcluster)  [unwired: 10 in]
      }
    }
    n83 = Wait (ms)(milliseconds to wait=u32 100) -> ()  [unwired: 1 out]
    n84 = Not(x=w206) -> (.not. x?=w190:bool)
    "Acquisition In Progress" <- w190
    n85 = call "Read GPIO Bank.vi"("fpga interface in"=w212, "gpio bank select"=w208, "error in (no error)"=w211) -> ("fpga interface out"=w199:refnum<k20>, "gpio bank output"=→"GPIO Bank Read":T9, "error out"=w200:errorcluster)  [unwired: 10 in]
    n86 = Bundle By Name(cluster=T1 {"ACQ. IN PROGRESS"=FALSE, "Array"=[]} ("Measurement Results"), "ACQ. IN PROGRESS"=w190, "Array"="Array") -> (w189:T1)
    n87 = call "Read Serial Input Channel Status.vi"("fpga interface in"=w199, "error in (no error)"=w200) -> ("fpga interface out"=w198:refnum<k20>, "error out"=w193:errorcluster)  [unwired: 11 in, 1 out]
    n88 = case shown="False" w187 {
      tunnel: w193 -> [w237 w238]
      tunnel: [w236 w238] -> w192
      tunnel: w191 -> [w235 _]
      tunnel: w189 -> [w234 _]
      frame False {
        n89 = call <vilib>:"Update Results.vi"("error in"=w237, "measurement results"=w234, "measure call context in"=w235) -> ("error out"=w236:errorcluster)  [unwired: 7 in, 1 out]
      }
      frame True {
      }
    }
    n90 = control-ref of="Channel Configurations"() -> (w202:refnum<vi>)
    n91 = call "Get Acq Raw Params.vi"("raw display notifier"=w201, "Channel Configurations"=w202, "error in (no error)"=w192) -> ("error out"=w203:errorcluster)  [unwired: 12 in]
  }
  n92 = control-ref of="Bytes Acquired (1st Channel)"() -> (w109:refnum<vi>)
  n93 = control-ref of="Bytes Acquired (2nd Channel)"() -> (w108:refnum<vi>)
  n94 = call "Image Display Loop.vi"("fpga interface in"=w63, "'stop' notifier"=w26, "rate references"=w75, "Ctl Refnum"=w1, "raw display notifier"=w22, "display references"=w88, "error in (no error)"=w64) -> ("error out"=w82:errorcluster)  [unwired: 8 in]
  n95 = Build Array(w109, w108) -> (w104:refnum<vi>[])
  n96 = call "Dispose Images.vi"("raw display notifier"=w22, "error in (no error)"=w82) -> ("error out"=w39:errorcluster)  [unwired: 13 in]
  n97 = call "LLP Packet Acquisition Loop.vi"("fpga interface in"=w63, "bytes acquired references"=w104, "Serial Channels"=w12, "tdms file directory"=w40, "display acquired packets"=w36, "error in"=w64, "log to disk"=w74, "num packets to read"=w35) -> ("number of packets acquired"=w103:i64[], "number of bytes acquired"=w72:i64[], "display data"=w73:string[][][], "error out"=w61:errorcluster)  [unwired: 4 in]
  n98 = flat-sequence {
    tunnel: "measurement configuration" -> [w257]
    tunnel: [w256] -> w3
    tunnel: "error in" -> [w255]
    tunnel: [w255] -> _
    frame #0 {
      n99 = Unbundle By Name(w257) -> ()  [unwired: 14 out]
      n100 = Bundle By Name(cluster=T1 {"ACQ. IN PROGRESS"=FALSE, "Array"=[]} ("Measurement Results"), "ACQ. IN PROGRESS"=FALSE) -> (w256:T1)
    }
  }
  n101 = Send Notification(notification=TRUE, notifier=w60) -> (notifier out=w59:refnum<notifier>, error out=w58:errorcluster)  [unwired: 1 in]
  n102 = Merge Errors(w39, w61, w58, w34, w33) -> (w19:errorcluster)
  n103 = Release Notifier(notifier=w59, force destroy? (F)=TRUE, error in (no error)=w19) -> (error out=w18:errorcluster)  [unwired: 2 out]
  n104 = Release Notifier(notifier=w20, force destroy? (F)=TRUE, error in (no error)=w19) -> (error out=w17:errorcluster)  [unwired: 2 out]
  n105 = Merge Errors(w18, w17) -> (w15:errorcluster)
  n106 = Index Array(array=w103) -> (element #1=w86:i64, element #2=w85:i64)  [unwired: 2 in]
  n107 = Index Array(array=w72) -> (element #1=w71:i64, element #2=w70:i64)  [unwired: 2 in]
  n108 = Index Array(array=w73) -> (element #1=w84:string[][], element #2=w83:string[][])  [unwired: 6 in]
  n109 = local write "TDMS File Directory"(w40) -> ()
  n110 = local write "Acquired Packets (2nd Channel)"(w83) -> ()
  n111 = local write "Acquired Packets (1st Channel)"(w84) -> ()
  n112 = local write "Bytes Acquired (1st Channel)"(w71) -> ()
  n113 = local write "Bytes Acquired (2nd Channel)"(w70) -> ()
  n114 = local write "Packets Logged (1st Channel)"(w86) -> ()
  n115 = local write "Packets Logged (2nd Channel)"(w85) -> ()
  n116 = call "Configure Serial Input Power Over Coax Source.vi"("fpga interface in"=w16, "serial input channels"=w12, "power over coax source"=w9, "error in (no error)"=w15) -> ("fpga interface out"=w7:refnum<k20>, "error out"=w8:errorcluster)  [unwired: 9 in, 1 out]
  n117 = call-poly <instrlib>:"Wait for PoC Safe to Disconnect.vi"("error in"=w8, "Timeout (ms)"=60000 ("Wait for Safe to Disconnect Timeout (ms)"), "Channels"=w12, "fpga interface in"=w7) -> ("error out"=w14:errorcluster, "fpga interface out"=w13:refnum<k20>)  [unwired: 6 in]
  n118 = xnode ("Close FPGA VI Reference")("FPGA VI Reference In"=w13, "error in"=w14) -> ("error out"=w5:errorcluster)
  n119 = call "Signal Measurement Complete.vi"("error in (no error)"=w5) -> ("error out"=w154:errorcluster, "done channel"=w155:T22)  [unwired: 9 in]
  n120 = call "Wait Until Cancelled or Complete.vi"("done channel"=w155, "error in (no error)"="error in", "measure call context in"="measure call context in") -> ("error out"=w153:errorcluster, "measure call context out"=→"measure call context out":refnum<class "Measure Call Context.lvclass">)  [unwired: 7 in]
  n121 = Merge Errors(w153, w154) -> (→"Error Out":errorcluster)
  "measurement results" <- w3
